vi "Test_Copy_Pixmap_to_Image_Greyscale.vi"(8 "error in (no error)":errorcluster, 11 "Test Case In":refnum<class "Image.lvclass">) -> (0 "error out":errorcluster, 3 "Test Case Out":refnum<class "Image.lvclass">)   [LabVIEW 2020, in "g_ar_toolkit.test.lvlib" / "Image.lvclass"]
uses:
  Image.lvclass
  Image.lvclass/Image.ctl
  g_ar_toolkit.image/g_ar_toolkit.image.lvlib
  g_ar_toolkit.image/CreateEmptyImageGreyscale.vi
  g_ar_toolkit.image/CopyPixmapToImageIgnoreMaskGreyscale.vi
  4993e8ee-a06a-463a-9684-69129f64d5ce.vi
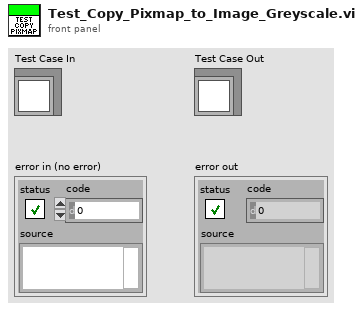
[diagram p1: front panel]
types:
  T1 = typedef "imagedata.ctl" = cluster{"image type":i32, "image depth":i32, "image":u8[], "mask":u8[], "colors":u32[], "Rectangle":cluster{"left":i16, "top":i16, "right":i16, "bottom":i16}}
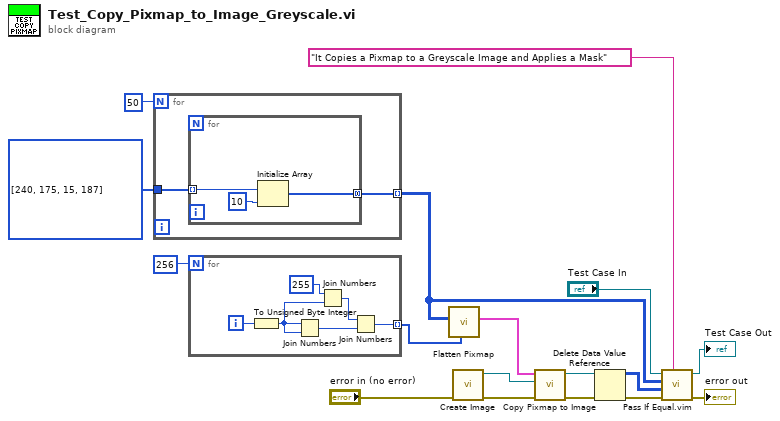
[diagram p0: block diagram]
diagram:
  n1 = for {
    N: 50 -> [_]
    tunnel: u8[] [240, 175, 15, 187] -> [w19]
    tunnel: [w18] -> w1 mode=indexing
    n2 = for {
      tunnel: w19 -> [w22] mode=indexing
      tunnel: [w21] -> w18 mode=concatenating
      n3 = Initialize Array(w22, 10 ("dimension size")) -> (w21:u8[])
    }
  }
  n4 = for {
    N: 256 -> [_]
    tunnel: [w23] -> w4 mode=indexing
    i -> [w28]
    n5 = To Unsigned Byte Integer(number=w28) -> (unsigned 8bit integer=w27:u8)
    n6 = Join Numbers(hi=w27, lo=w27) -> ((hi.lo)=w26:u16)
    n7 = Join Numbers(hi=u8 255, lo=w27) -> ((hi.lo)=w25:u16)
    n8 = Join Numbers(hi=w25, lo=w26) -> ((hi.lo)=w23:u32)
  }
  n9 = call <vilib>:"Flatten Pixmap.vi"("colors"=w4, "8-bit pixmap"=w1) -> ("image data"=w3:T1)  [unwired: 9 in]
  n10 = call-poly "Create Image.vi"("error in (no error)"="error in (no error)") -> ("error out"=w11:errorcluster, "New Greyscale Image"=w10:refnum<data-value>)  [unwired: 9 in]
  n11 = call-poly "Copy Pixmap to Image.vi"("error in (no error)"=w11, "Greyscale Image Destination"=w10, "Pixmap Image Data"=w3) -> ("error out"=w9:errorcluster, "Greyscale Image Destination (duplicate)"=w8:refnum<data-value>)  [unwired: 7 in]
  n12 = Delete Data Value Reference(data value reference=w8, error in=w9) -> (data value=w2:u8[][], error out=w12:errorcluster)
  n13 = call "Pass If Equal.vim"("Description"="It Copies a Pixmap to a Greyscale Image and Applies a Mask", "error in (no error)"=w12, "Actual"=w2, "Expected"=w1, "LUnit Test Case In"="Test Case In") -> ("error out"=→"error out":errorcluster, "LUnit Test Case Out"=→"Test Case Out":refnum<class "Image.lvclass">)  [unwired: 5 in]
